vi "Set Timeout.vi"(8 "error in (no error)":errorcluster, 10 "Timeout Period in ms (-1, never)":i32=-1, 11 "_State Machine Actor in":refnum<class "_State Machine Actor.lvclass">) -> (0 "error out":errorcluster, 3 "_State Machine Actor out":refnum<class "_State Machine Actor.lvclass">)   [LabVIEW 2024]
uses:
  _State Machine Actor.lvclass
  _State Machine Actor Messages/Timeout Msg/Timeout Msg.lvclass
  <vilib>/ActorFramework/Actor/Actor.lvclass/Actor.ctl
  <vilib>/ActorFramework/Message Enqueuer/Message Enqueuer.lvclass/Message Enqueuer.ctl
  _State Machine Actor.lvclass/_State Machine Actor.ctl
  <vilib>/ActorFramework/Message Enqueuer/Init from Existing Queue.vi
  <vilib>/ActorFramework/Message Enqueuer/Message Enqueuer.lvclass
  <vilib>/ActorFramework/Actor/Actor.lvclass
  C:/Program Files (x86)/National Instruments/LabVIEW 2024/vi.lib/ActorFramework/Message/Message.lvclass
  C:/Users/uspoaotto/OneDrive - Oregon Tool/Desktop/working copies/stateMachineActor/src/_State Machine Actor/_State Machine Actor Messages/Timeout Msg/Timeout Msg.lvclass
  C:/Program Files (x86)/National Instruments/LabVIEW 2024/vi.lib/ActorFramework/Actor/Actor.lvclass
  C:/Users/uspoaotto/OneDrive - Oregon Tool/Desktop/working copies/stateMachineActor/src/_State Machine Actor/_State Machine Actor/_State Machine Actor.lvclass
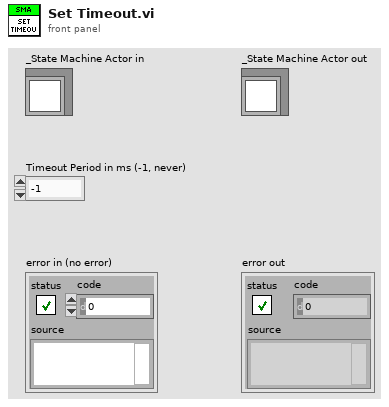
[diagram p1: front panel]
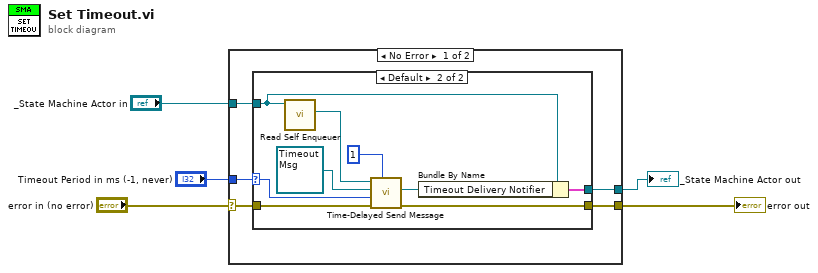
[diagram p0: block diagram]
diagram:
  n1 = case shown="No Error" "error in (no error)" {
    selector: "error in (no error)" -> [w6 w23]
    tunnel: [w7 w23] -> w4
    tunnel: [w8 w22] -> w2
    tunnel: "_State Machine Actor in" -> [w10 w22]
    tunnel: "Timeout Period in ms (-1, never)" -> [w9 _]
    frame No Error {
      n2 = case shown="Default" w9 {
        selector: w9 -> [_ w20]
        tunnel: [w11 w18] -> w8
        tunnel: [w12 w17] -> w7
        tunnel: w10 -> [w11 w13]
        tunnel: w6 -> [w12 w14]
        frame -1 {
        }
        frame Default {
          n3 = call <vilib>:"Read Self Enqueuer.vi"("Actor"=w13) -> ("Self Enqueuer"=w15:refnum<class "Message Enqueuer.lvclass">)  [unwired: 10 in]
          n4 = call <vilib>:"Time-Delayed Send Message.vi"("# Copies (0 = infinite repeat)"=u32 1, "error in (no error)"=w14, "Milliseconds To Wait"=w20, "Message"=refnum<class "Timeout Msg.lvclass"> refnum ("_State Machine Actor.lvlib:Timeout Msg.lvclass"), "Message Enqueuer"=w15) -> ("error out"=w17:errorcluster, "Delivery Notifier"=w19:refnum<notifier>)  [unwired: 5 in]
          n5 = Bundle By Name(cluster=w13, "Timeout Delivery Notifier"=w19) -> (w18:cluster{})
        }
      }
    }
    frame Error {
    }
  }
  "error out" <- w4
  "_State Machine Actor out" <- w2
